vi "NUC-T判定.vi"(2 "高低增益对比数据":u16=4048 format="%.0x", 3 "data in":u16[](array[numeric])) -> (7 "result":bool)   [LabVIEW 2016]
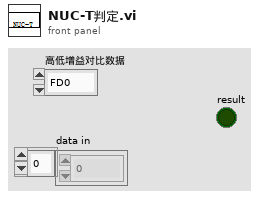
[diagram p1: front panel]
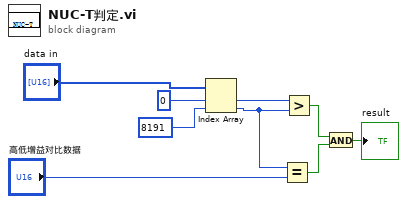
[diagram p0: block diagram]
diagram:
  n1 = Index Array(array="data in", index #1=0 ("index"), index #2=8191 ("index")) -> (element #1=w4:u16, element #2=w3:u16)
  n2 = Equal?(x=w3, y="高低增益对比数据") -> (x = y?=w1:bool)
  n3 = Greater?(x=w4, y=w3) -> (0:w2:bool)
  n4 = And(x=w2, y=w1) -> (x .and. y?=→"result":bool)
